vi "GetAttributeViBoolean.vi"(8 "error in (no error)":errorcluster {"code" format="%.0x"}, 9 "AttributeID":u32(ring)=1150001 items=["CHANNEL_AVERAGING"=1150001, "CHANNEL_CORRECTION"=1150003, "CHANNEL_IS_SWEEP_COMPLETE"=1150115, "CHANNEL_MEASUREMENT_LIMIT_ENABLE"=1150018, "CHANNEL_MEASUREMENT_LIMIT_IS_PASSING"=1150019, "CHANNEL_MEASUREMENT_MARKER_ENABLED"=1150022, "CHANNEL_MEASUREMENT_MARKER_MARKER_TRACK_ENABLED"=1150023, "CHANNEL_MEASUREMENT_SMOOTHING"=1150015, "CHANNEL_MEASUREMENT_TIME_DOMAIN_COUPLING_STATE"=1150136, "CHANNEL_MEASUREMENT_TIME_DOMAIN_GATING_ENABLE"=1150139, "CHANNEL_MEASUREMENT_TIME_DOMAIN_TRANSFORM_ENABLE"=1150146, "CHANNEL_MEASUREMENT_TRACE_ENABLE_TRACE_MAX"=1150182, "CHANNEL_PORT_EXTENSION_STATUS"=1150008, "CHANNEL_SOURCEPOWER_COUPLING"=1150031, "CHANNEL_SWEEP_TIME_AUTO"=1150011, "DISPLAY_ENABLED"=1150036, "GUIDED_CALIBRATION_ADVANCED_E_CAL_AUTO_ORIENTATION"=1150116, "GUIDED_CALIBRATION_CALIBRATION_STEP_IS_ACQUISITION_COMPLETE"=1150155, "GUIDED_CALIBRATION_CALIBRATION_STEP_IS_COMPLETED"=1150156, "GUIDED_CALIBRATION_CALIBRATION_STEP_IS_OPTIONAL"=1150157, "IS_OPERATION_COMPLETE"=1150165, "SIMULATE"=1050005, "SYSTEM_POWER_ENABLED"=1150184, "SYSTEM_TRACE_ENABLED"=1150041, "WINDOW_STATE"=1150183, "WINDOW_TITLE_STATE"=1150132], 10 "RepCapIdentifier":string, 11 "instrument handle":refnum<k15>) -> (0 "error out":errorcluster {"code" format="%.0x"}, 2 "AttributeValue":bool, 3 "instrument handle out":refnum<k15>)   [LabVIEW 2014, in "Agilent NA.lvlib"]
doc: "Gets a Boolean attribute from the instrument driver.\nThe following Attributes are supported:\n\nCHANNEL_AVERAGING\nCHANNEL_CORRECTION\nCHANNEL_IS_SWEEP_COMPLETE\nCHANNEL_MEASUREMENT_LIMIT_ENABLE\nCHANNEL_MEASUREMENT_LIMIT_IS_PASSING\nCHANNEL_MEASUREMENT_MARKER_ENABLED\nCHANNEL_MEASUREMENT_MARKER_MARKER_TRACK_ENABLED\nCHANNEL_MEASUREMENT_SMOOTHING\nCHANNEL_MEASUREMENT_TIME_DOMAIN_COUPLING_STATE\nCHANNEL_MEASUREMENT_TIME_DOMAIN_GATING_ENABLE\nCHANNEL_MEASUREMENT_TIME_DOMAIN_TRANSFORM_ENABLE\nCHANNEL_MEASUREMENT_TRACE_ENABLE_TRACE_MAX\nCHANNEL_PORT_EXTENSION_STATUS\nCHANNEL_SOURCEPOWER_COUPLING\nCHANNEL_SWEEP_TIME_AUTO\nDISPLAY_ENABLED\nGUIDED_CALIBRATION_ADVANCED_E_CAL_AUTO_ORIENTATION\nGUIDED_CALIBRATION_CALIBRATION_STEP_IS_ACQUISITION_COMPLETE\nGUIDED_CALIBRATION_CALIBRATION_STEP_IS_COMPLETED\nGUIDED_CALIBRATION_CALIBRATION_STEP_IS_OPTIONAL\nIS_OPERATION_COMPLETE\nSIMULATE\nSYSTEM_POWER_ENABLED\nSYSTEM_TRACE_ENABLED\nWINDOW_STATE\nWINDOW_TITLE_STATE"
uses:
  Agilent NA.lvlib
  AgNA.dll
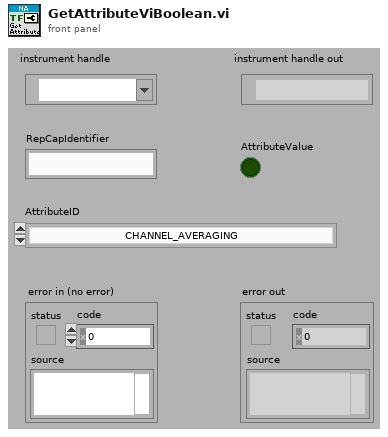
[diagram p1: front panel]
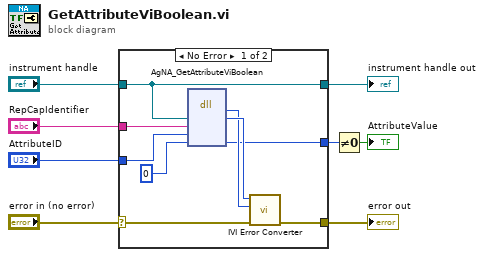
[diagram p0: block diagram]
diagram:
  n1 = case shown="No Error" "error in (no error)" {
    selector: "error in (no error)" -> [w15 w19]
    tunnel: [w14 w19] -> w8
    tunnel: "RepCapIdentifier" -> [w13 _]
    tunnel: "AttributeID" -> [w12 _]
    tunnel: [w10 _] -> w3
    tunnel: [w9 w18] -> w2
    tunnel: "instrument handle" -> [w9 w18]
    frame No Error {
      n2 = dll-call lib="AgNA**.dll" fn="AgNA_GetAttributeViBoolean"("Vi"=w9, "RepCapIdentifier"=w13, "AttributeID"=w12, "AttributeValue"=i16 0) -> ("return type"=w16:i32, "Vi"=w17:u32, "AttributeValue"=w10:i16)  [unwired: 5 in, 2 out]
      n3 = call "IVI Error Converter.vi"("error in (no error)"=w15, "IVI error code (0)"=w16, "instrument handle"=w17) -> ("error out"=w14:errorcluster)  [unwired: 7 in, 1 out]
    }
    frame Error {
    }
  }
  "error out" <- w8
  "instrument handle out" <- w2
  n4 = Not Equal To 0?(x=w3) -> (x != 0?=→"AttributeValue":bool)
